vi "mav_global_var.vi"() -> ()   [LabVIEW 2023]
panel:
  out "ATTITUDE #30":T1
  in  "stop":bool
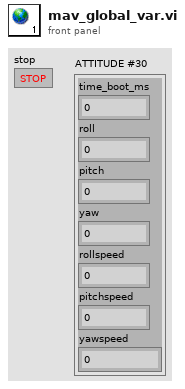
[diagram p1: front panel]
types:
  T1 = cluster{"time_boot_ms":u32, "roll":sgl, "pitch":sgl, "yaw":sgl, "rollspeed":sgl, "pitchspeed":sgl, "yawspeed":sgl}
diagram:
